vi "PDW gen.vi"(5 "num of channels":i32, 7 "niqiest freqency":dbl=125000000.0 format="%#_13g", 8 "D.C":dbl=1.5 format="%#_13g", 9 "pulse amplitude":dbl format="%#_13g", 10 "pulse duration":dbl=0.1 format="%#_13g", 11 "frequency list":dbl[](array[numeric])=[60000000.0, 70000000.0, 130000000.0, 260000000.0]) -> (2 "niqiest band":dbl[](array[numeric])=[0.0, 1.0, 2.0], 3 "PDWs on channels":cluster{T1[]}[](array[cluster]))   [LabVIEW 2021]
uses:
  CTL/PDW_lv2.ctl
  CTL/mode_type.ctl
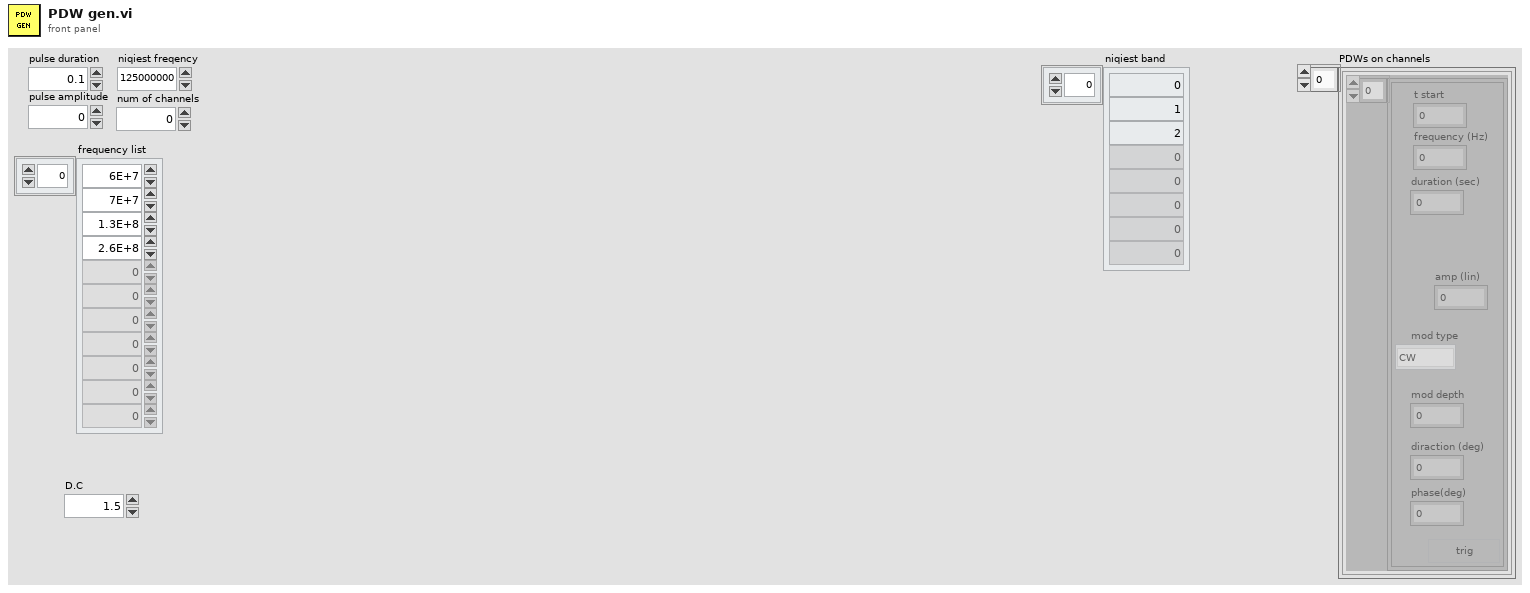
[diagram p1: front panel]
types:
  T1 = typedef "PDW_lv2.ctl" = cluster{"t start":dbl, "frequency (Hz)":dbl, "duration (sec)":dbl, "mod type":T2, "mod depth":dbl, "trig":bool, "amp (lin)":dbl, "diraction (deg)":dbl, "phase(deg)":dbl}
  T2 = typedef "mode_type.ctl" = enum8{"CW", "from memory 1", "NC - cw", "LFM", "BPSK", "QPSK"}
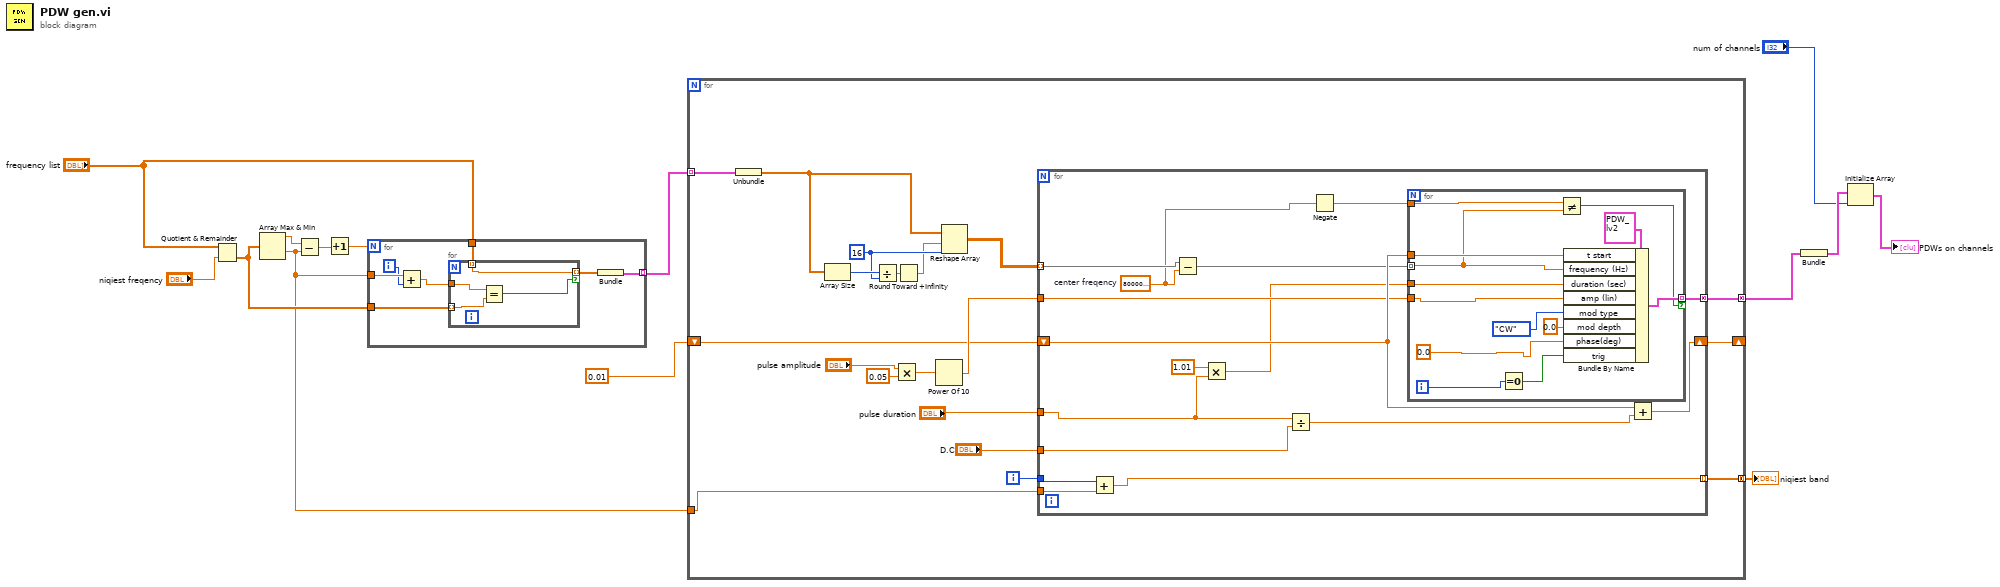
[diagram p0: block diagram]
diagram:
  n1 = Quotient & Remainder(x="frequency list", y="niqiest freqency") -> (floor(x/y)=w12:dbl[])  [unwired: 1 out]
  n2 = Array Max & Min(array=w12) -> (max value=w13:dbl, min value=w8:dbl)  [unwired: 2 out]
  n3 = Subtract(x=w13, y=w8) -> (x-y=w6:dbl)
  n4 = Increment(x=w6) -> (x+1=w5:dbl)
  n5 = for {
    N: w5 -> [_]
    tunnel: w8 -> [w21]
    tunnel: w12 -> [w19]
    tunnel: "frequency list" -> [w17]
    tunnel: [w15] -> w10 mode=indexing
    i -> [w20]
    n6 = Add(x=w21, y=w20) -> (x+y=w18:dbl)
    n7 = for {
      tunnel: w19 -> [w25] mode=indexing
      tunnel: w18 -> [w24]
      tunnel: [w23] -> w16 mode=indexing if=w22
      tunnel: w17 -> [w23] mode=indexing
      n8 = Equal?(x=w24, y=w25) -> (x = y?=w22:bool)
    }
    n9 = Bundle(w16) -> (w15:cluster{dbl[]})  [unwired: 1 in]
  }
  n10 = for {
    tunnel: [w38] -> w4 mode=concatenating
    tunnel: w10 -> [w32] mode=indexing
    shift-right: [w30] -> _
    shift-left: 0.01 -> [w29]
    tunnel: [w27] -> w7 mode=concatenating
    tunnel: w8 -> [w26]
    i -> [w28]
    w36 = 16 ("dimension size")
    n11 = Unbundle(w32) -> (w31:dbl[])
    n12 = Array Size(array=w31) -> (size(s)=w37:i32)
    n13 = Divide(x=w37, y=w36) -> (x/y=w35:dbl)
    n14 = Multiply(x="pulse amplitude", y=0.05) -> (x*y=w42:dbl)
    n15 = Round Toward +Infinity(x=w35) -> (ceil(x): smallest int >= x=w34:dbl)
    n16 = Power Of 10(x=w42) -> (10^x=w39:dbl)
    n17 = Reshape Array(w31, w34, w36) -> (w44:dbl[][])
    n18 = for {
      tunnel: w44 -> [w57] mode=indexing
      tunnel: "pulse duration" -> [w53]
      shift-right: [w60] -> w30
      shift-left: w29 -> [w58]
      tunnel: w39 -> [w55]
      tunnel: [w54] -> w38 mode=concatenating
      tunnel: "D.C" -> [w50]
      tunnel: w28 -> [w48]
      tunnel: [w47] -> w27 mode=indexing
      tunnel: w26 -> [w49]
      w46 = 800000000.0  # center freqency
      n19 = Add(x=w48, y=w49) -> (x+y=w47:dbl)
      n20 = Subtract(x=w57, y=w46) -> (x-y=w56:dbl[])
      n21 = Multiply(x=1.01, y=w53) -> (x*y=w51:dbl)
      n22 = Divide(x=w53, y=w50) -> (x/y=w59:dbl)
      n23 = Negate(x=w46) -> (-x=w45:dbl)
      n24 = for {
        tunnel: w58 -> [w72]
        tunnel: w51 -> [w71]
        tunnel: w56 -> [w65] mode=indexing
        tunnel: w55 -> [w62]
        tunnel: [w69] -> w54 mode=indexing if=w64
        tunnel: w45 -> [w63]
        i -> [w66]
        n25 = Equal To 0?(x=w66) -> (x = 0?=w67:bool)
        n26 = Not Equal?(x=w63, y=w65) -> (x != y?=w64:bool)
        n27 = Bundle By Name(cluster=T1 {"t start"=0.0, "frequency (Hz)"=0.0, "duration (sec)"=0.0, "mod type"=enum."CW", "mod depth"=0.0, "trig"=FALSE, "amp (lin)"=0.0, "diraction (deg)"=0.0, "phase(deg)"=0.0}, "t start"=w72, "frequency (Hz)"=w65, "duration (sec)"=w71, "amp (lin)"=w62, "mod type"=mode_type."CW", "mod depth"=0.0, "phase(deg)"=0.0 ("element"), "trig"=w67) -> (w69:T1)
      }
      n28 = Add(x=w58, y=w59) -> (x+y=w60:dbl)
    }
  }
  "niqiest band" <- w7
  n29 = Bundle(w4) -> (w3:cluster{T1[]})  [unwired: 1 in]
  n30 = Initialize Array(w3, "num of channels") -> (→"PDWs on channels":cluster{T1[]}[])
